vi "Get Object Offset.vi"(6 "Side":T1=enum."right", 8 "error in":errorcluster, 11 "Label":string="Large Gear") -> (0 "error out":errorcluster, 1 "GraspClose":bool, 2 "XYZOAT":T2, 3 "T":T3 format="%.3f")   [LabVIEW 2013]
uses:
  <vilib>/Analysis/Matrix/Datatypes/RealMatrix.ctl
  ROS/Code/SubVIs/BaxterSide.ctl
  Arm Globals.vi
  <vilib>/Utility/config.llb/Read Key (String).vi
  <vilib>/Utility/config.llb/Read Key (Boolean).vi
  <vilib>/Utility/config.llb/NI_LVConfig.lvlib
  <vilib>/Analysis/Matrix/NI_Matrix.lvlib
panel:
  # "Y"
  # "X"
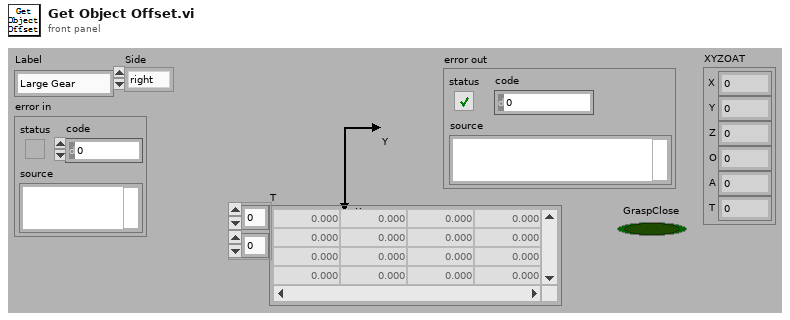
[diagram p1: front panel]
types:
  T1 = typedef "BaxterSide.ctl" = enum16{"left", "right"}
  T2 = cluster{"X":dbl, "Y":dbl, "Z":dbl, "O":dbl, "A":dbl, "T":dbl}
  T3 = typedef "NI_Matrix.lvlib/RealMatrix.ctl" = dbl[][]
  T4 = typedef "NI_LVConfig.lvlib/Config Data RefNum.ctl" = refnum<k1>
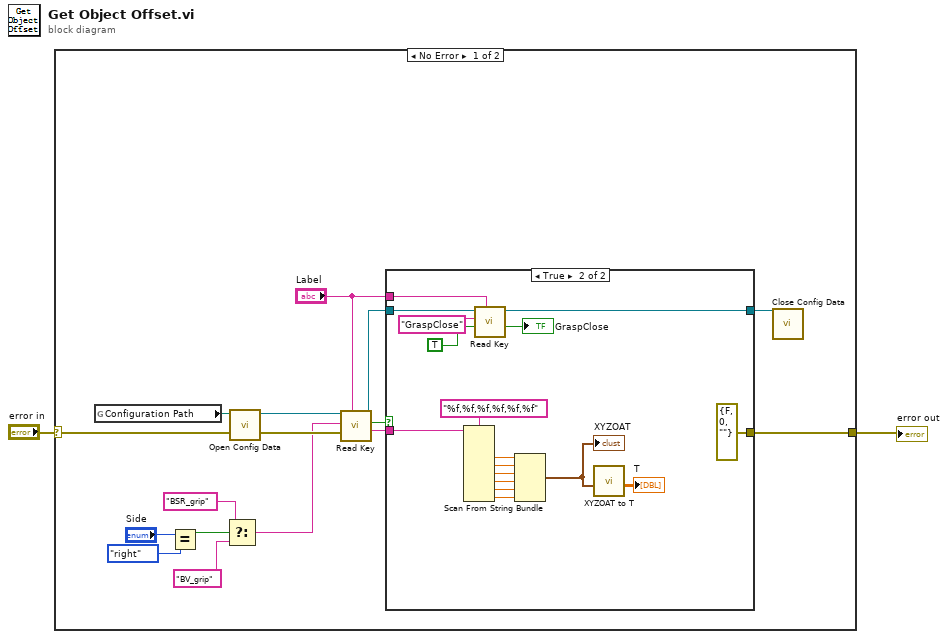
[diagram p0: block diagram]
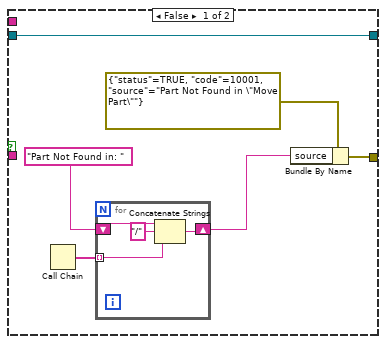
[diagram p2: hidden frame]
diagram:
  n1 = case shown="No Error" "error in" {
    selector: "error in" -> [w16 w45]
    tunnel: [w15 w45] -> w1
    frame No Error {
      n2 = global read "Arm Globals.vi" "Configuration Path"() -> (w9:path)
      n3 = Equal?(x="Side", y=BaxterSide."right") -> (x = y?=w6:bool)
      n4 = Select(t="BSR_grip", s=w6, f="BV_grip") -> (s? t:f=w4:string)
      n5 = call <vilib>:"Open Config Data.vi"("configuration file path"=w9) -> ("refnum"=w14:T4)  [unwired: 8 in, 2 out]
      n6 = call-poly <vilib>:"Read Key.vi"("section"="Label", "error in (no error)"=w16, "key"=w4, "refnum"=w14) -> ("value"=w17:string, "found?"=w13:bool, "refnum out"=w12:T4)  [unwired: 4 in, 1 out]
      n7 = case shown="True" w13 {
        tunnel: w17 -> [_ w36]
        tunnel: [w21 errorcluster {"status"=FALSE, "code"=0, "source"=""} ("error out")] -> w15
        tunnel: w12 -> [w18 w42]
        tunnel: [w18 w41] -> w11
        tunnel: "Label" -> [_ w40]
        frame False {
          n8 = Call Chain() -> (call chain=w22:string[])
          n9 = for {
            tunnel: w22 -> [w25] mode=indexing
            shift-right: [w27] -> w20
            shift-left: "Part Not Found in: " ("source") -> [w26]
            n10 = Concatenate Strings(w26, "/" ("string"), w25) -> (w27:string)
          }
          n11 = Bundle By Name(cluster=errorcluster {"status"=TRUE, "code"=10001, "source"="Part Not Found in \"Move Part\""} ("error out"), "source"=w20) -> (w21:errorcluster)
        }
        frame True {
          n12 = Scan From String(format string="%f,%f,%f,%f,%f,%f", input string=w36) -> (output 1=w34:dbl, output 2=w33:dbl, output 3=w32:dbl, output 4=w31:dbl, output 5=w30:dbl, output 6=w29:dbl)  [unwired: 8 in, 3 out]
          n13 = call-poly <vilib>:"Read Key.vi"("section"=w40, "default value"=TRUE, "key"="GraspClose", "refnum"=w42) -> ("value"=→"GraspClose":bool, "refnum out"=w41:T4)  [unwired: 4 in, 2 out]
          n14 = Bundle(w34, w33, w32, w31, w30, w29) -> (w28:cluster{dbl, dbl, dbl, dbl, dbl, dbl})  [unwired: 1 in]
          "XYZOAT" <- w28
          n15 = call "XYZOAT to T.vi"("XYZOAT"=w28) -> ("T"=→"T":T3)  [unwired: 10 in]
        }
      }
      n16 = call <vilib>:"Close Config Data.vi"("refnum"=w11) -> ()  [unwired: 9 in, 2 out]
    }
    frame Error {
    }
  }
  "error out" <- w1
